vi "Connect.vi"(8 "error in (no error)":errorcluster, 11 "F4T in":refnum<class "F4T.lvclass">) -> (0 "error out":errorcluster, 3 "F4T out":refnum<class "F4T.lvclass">)   [LabVIEW 2018, in "F4T.lvlib" / "F4T.lvclass"]
uses:
  F4T.lvclass
  Custom Controls/Control Data.ctl
  F4T.lvclass/F4T.ctl
  PPLs/Temp Chamber/Parent/Temp Chamber.lvlibp/Temp Chamber.lvclass
  C:/Projects/LabVIEW/PPLs/Temp Chamber/Parent/Temp Chamber.lvlibp/Temp Chamber.lvclass
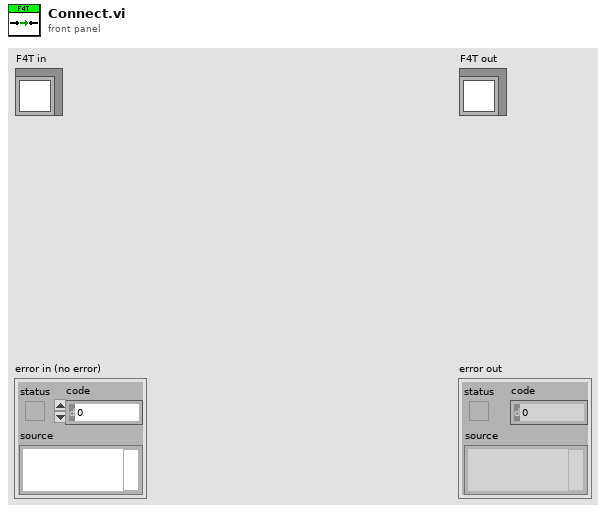
[diagram p1: front panel]
types:
  T1 = typedef "F4T.lvlib/F4T.lvclass/Control Data.ctl" = cluster{"DeviceType ":u32, "Zone":u32}
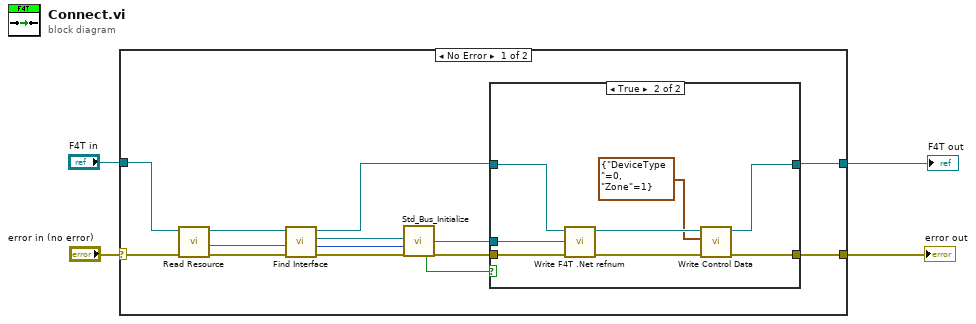
[diagram p0: block diagram]
diagram:
  n1 = case shown="No Error" "error in (no error)" {
    selector: "error in (no error)" -> [w17 w29]
    tunnel: "F4T in" -> [w18 w30]
    tunnel: [w12 w30] -> w2
    tunnel: [w13 w29] -> w1
    frame No Error {
      n2 = call "Read Resource.vi"("error in (no error)"=w17, "Temp Chamber in"=w18) -> ("error out"=w11:errorcluster, "Resource"=w10:refnum<visa-resource-name>, "Temp Chamber out"=w9:refnum<class "F4T.lvclass">)  [unwired: 7 in]
      n3 = call "Find Interface.vi"("error in (no error)"=w11, "Resource"=w10, "F4T in"=w9) -> ("error out"=w5:errorcluster, "InterfaceType"=w6:i32, "Resource out"=w7:refnum<visa-resource-name>, "F4T out"=w8:refnum<class "F4T.lvclass">)  [unwired: 5 in]
      n4 = call <instrlib>:"Std_Bus_Initialize.vi"("Communications Port"=w7, "InterfaceType"=w6, "error in (no error)"=w5) -> ("IsConnected"=w16:bool, "ILabVIEW"=w14:refnum<k24>, "error out"=w15:errorcluster)  [unwired: 14 in]
      n5 = case shown="True" w16 {
        tunnel: w15 -> [w19 w28]
        tunnel: w14 -> [_ w27]
        tunnel: w8 -> [w20 w26]
        tunnel: [w19 w23] -> w13
        tunnel: [w20 w22] -> w12
        frame False {
        }
        frame True {
          n6 = call "Write F4T .Net refnum.vi"("error in (no error)"=w28, "F4T .Net refnum"=w27, "F4T in"=w26) -> ("error out"=w25:errorcluster, "F4T out"=w24:refnum<class "F4T.lvclass">)  [unwired: 7 in]
          n7 = call "Write Control Data.vi"("error in (no error)"=w25, "Control Data"=T1 {"DeviceType "=0, "Zone"=1}, "F4T in"=w24) -> ("error out"=w23:errorcluster, "F4T out"=w22:refnum<class "F4T.lvclass">)  [unwired: 7 in]
        }
      }
    }
    frame Error {
    }
  }
  "error out" <- w1
  "F4T out" <- w2
